vi "AlAs_GaAs_SL3.vi"(2 "Debug Mode":bool, 3 "Elapsed Time (s)":dbl, 4 "State":enum16{"Edit", "Start", "Run", "End", "Idle"}(ring), 5 "Argument List In":string[](array[string])) -> (0 "Status Out":string, 1 "Argument List Out":string[](array[string]))   [LabVIEW 2011]
doc: "This VI oscillates the flow of Gallium in a square wave according to the \"Period\" and \"Amplitude\" parameters. See the API Programming Guide for more details."
panel:
  out "tTot(s)":dbl
  in  "periods":dbl
  in  "tGa (s)":dbl
  in  "Ga flow (sccm)":dbl
  out "Timer":dbl
  out "Previous Time":dbl
  in  "tAl (s)":dbl
  in  "Al flow (sccm)":dbl
  in  "Cancel":bool
  in  "OK":bool
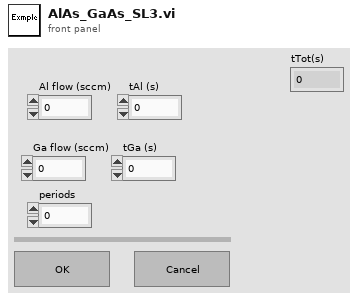
[diagram p1: front panel]
types:
  T1 = enum16{"Discrete", "Continuous", "Instantaneous"}
  T2 = enum32{"Invalid", "Default", "Floating", "Floating/Auto-Hide", "Modal"}
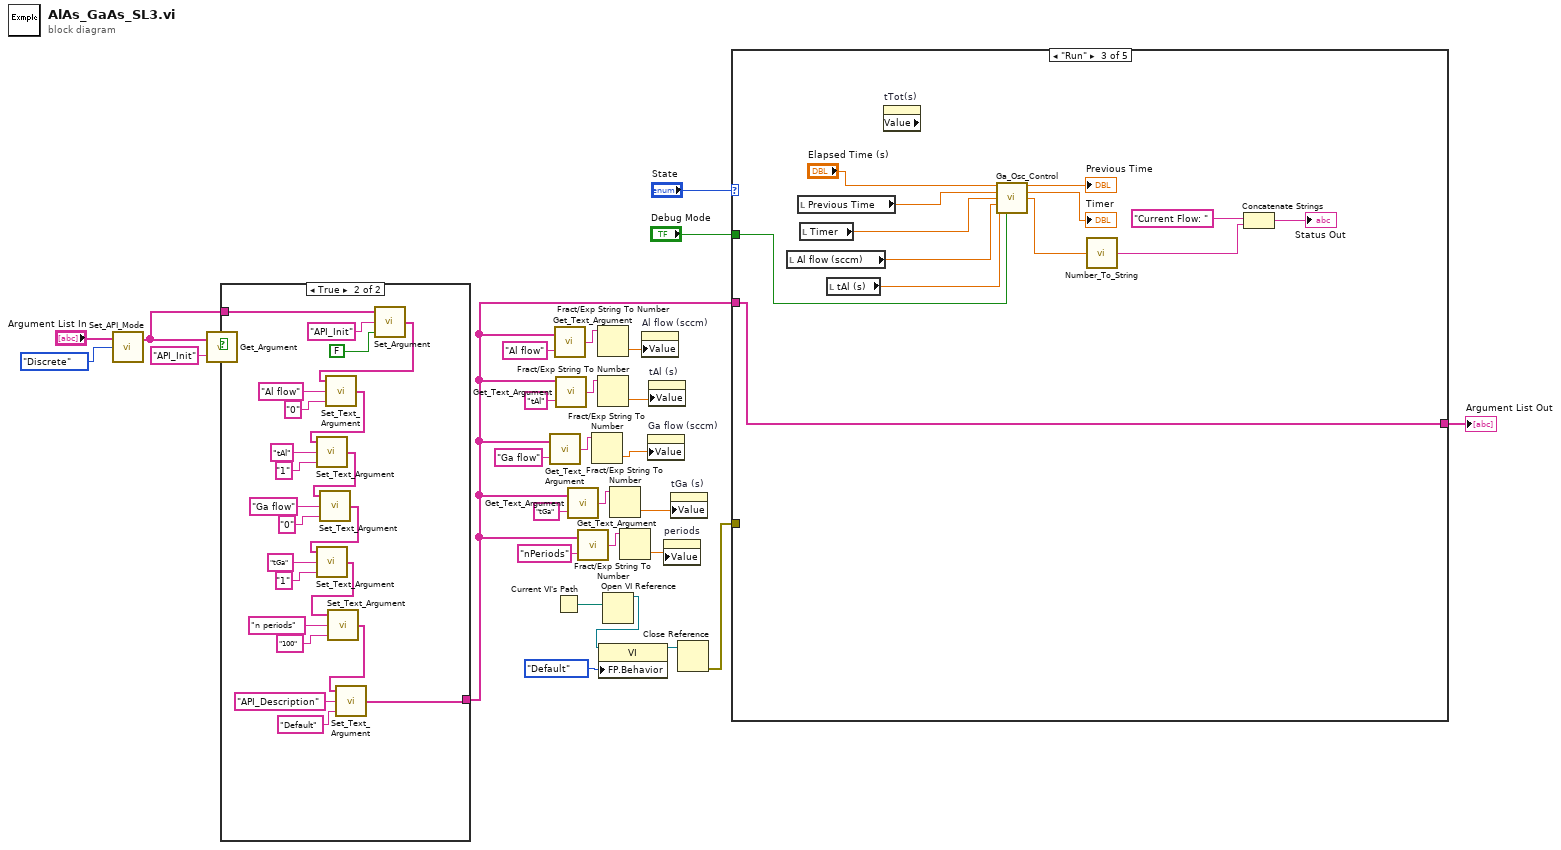
[diagram p0: block diagram]
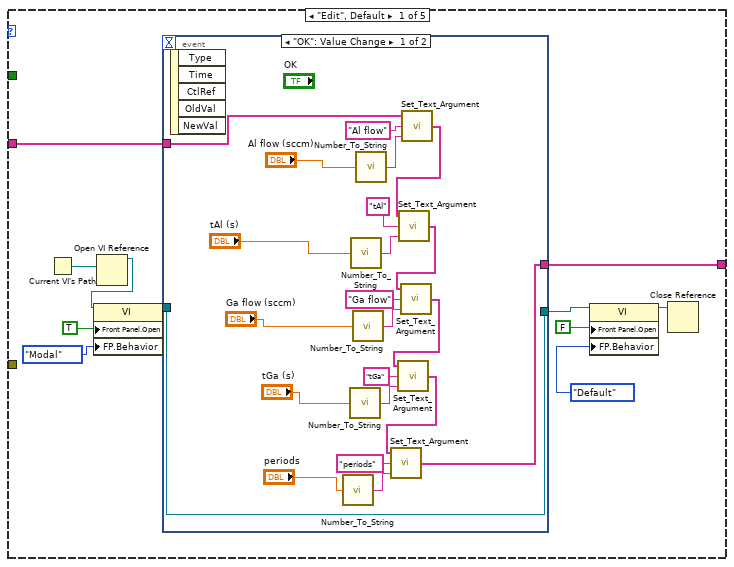
[diagram p3: hidden frame]
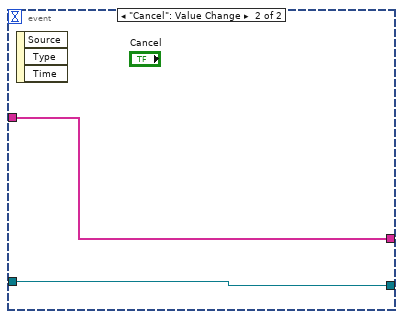
[diagram p4: hidden frame]
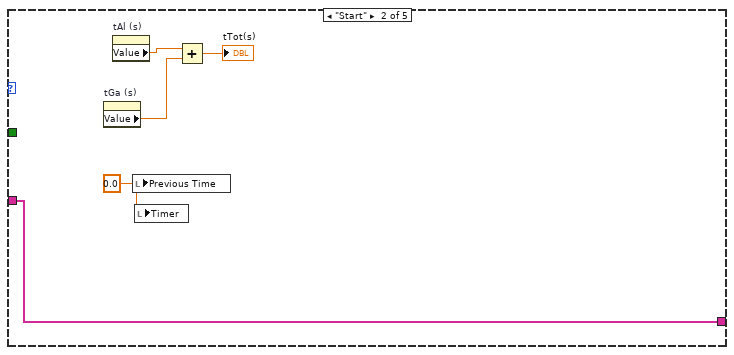
[diagram p5: hidden frame]
diagram:
  n1 = call "Set_API_Mode.vi"("API Mode"=T1."Discrete", "Argument List In"="Argument List In") -> ("Argument List Out"=w16:string[])  [unwired: 2 out]
  n2 = call "Get_Argument.vi"("Argument"="API_Init", "Argument List"=w16) -> ("Enabled"=w17:bool)
  n3 = case shown="True" w17 {
    tunnel: w16 -> [w30 w52]
    tunnel: [w30 w48] -> w6
    frame False {
    }
    frame True {
      n4 = call "Set_Argument.vi"("Enable"=FALSE, "Argument"="API_Init", "Argument List In"=w52) -> ("Argument List Out"=w31:string[])
      n5 = call "Set_Text_Argument.vi"("Text"="0", "Argument"="Al flow", "Argument List In"=w31) -> ("Argument List Out"=w32:string[])
      n6 = call "Set_Text_Argument.vi"("Text"="1", "Argument"="tAl", "Argument List In"=w32) -> ("Argument List Out"=w33:string[])
      n7 = call "Set_Text_Argument.vi"("Text"="0", "Argument"="Ga flow", "Argument List In"=w33) -> ("Argument List Out"=w34:string[])
      n8 = call "Set_Text_Argument.vi"("Text"="1", "Argument"="tGa", "Argument List In"=w34) -> ("Argument List Out"=w35:string[])
      n9 = call "Set_Text_Argument.vi"("Text"="100", "Argument"="n periods", "Argument List In"=w35) -> ("Argument List Out"=w36:string[])
      n10 = call "Set_Text_Argument.vi"("Text"="Default", "Argument"="API_Description", "Argument List In"=w36) -> ("Argument List Out"=w48:string[])
    }
  }
  n11 = call "Get_Text_Argument.vi"("Argument"="Ga flow", "Argument List"=w6) -> ("Text"=w11:string)
  n12 = Current VI's Path() -> (path=w25:path)
  n13 = call "Get_Text_Argument.vi"("Argument"="Al flow", "Argument List"=w6) -> ("Text"=w14:string)
  n14 = call "Get_Text_Argument.vi"("Argument"="tAl", "Argument List"=w6) -> ("Text"=w13:string)
  n15 = call "Get_Text_Argument.vi"("Argument"="tGa", "Argument List"=w6) -> ("Text"=w9:string)
  n16 = call "Get_Text_Argument.vi"("Argument"="nPeriods", "Argument List"=w6) -> ("Text"=w7:string)
  n17 = Fract/Exp String To Number(string=w11) -> (number=w3:dbl)  [unwired: 4 out]
  n18 = Fract/Exp String To Number(string=w14) -> (number=w5:dbl)  [unwired: 4 out]
  n19 = Fract/Exp String To Number(string=w13) -> (number=w4:dbl)  [unwired: 4 out]
  n20 = Open VI Reference(vi path=w25) -> (vi reference=w24:refnum<vi>)  [unwired: 1 in, 5 out]
  n21 = property class="VI"(reference=w24, "FP.Behavior"=T2."Default" ("Front Panel Window:Behavior")) -> (reference out=w22:refnum<vi>)  [unwired: 1 in, 1 out]
  n22 = Fract/Exp String To Number(string=w9) -> (number=w2:dbl)  [unwired: 4 out]
  n23 = Fract/Exp String To Number(string=w7) -> (number=w1:dbl)  [unwired: 4 out]
  n24 = property on="Al flow (sccm)" class="DigNum (strict)"("Value"=w5) -> ()  [unwired: 2 in, 2 out]
  n25 = property on="Ga flow (sccm)" class="DigNum (strict)"("Value"=w3) -> ()  [unwired: 2 in, 2 out]
  n26 = property on="tAl (s)" class="DigNum (strict)"("Value"=w4) -> ()  [unwired: 2 in, 2 out]
  n27 = property on="periods" class="DigNum (strict)"("Value"=w1) -> ()  [unwired: 2 in, 2 out]
  n28 = property on="tGa (s)" class="DigNum (strict)"("Value"=w2) -> ()  [unwired: 2 in, 2 out]
  n29 = Close Reference(reference=w22) -> (error out=w21:errorcluster)  [unwired: 1 in]
  n30 = case shown="\"Run\"" "State" {
    tunnel: [w63 w92 w103 w107 w108] -> w28
    tunnel: w6 -> [w62 w92 w103 w107 w108]
    tunnel: "Debug Mode" -> [_ _ w93 w106 _]
    tunnel: w21 -> [_ _ _ _ _]
    frame "Edit", Default {
      n31 = Current VI's Path() -> (path=w57:path)
      n32 = Open VI Reference(vi path=w57) -> (vi reference=w56:refnum<vi>)  [unwired: 1 in, 5 out]
      n33 = property class="VI"(reference=w56, "Front Panel.Open"=TRUE ("Front Panel Window:Open"), "FP.Behavior"=T2."Modal" ("Front Panel Window:Behavior")) -> (reference out=w60:refnum<vi>)  [unwired: 1 in, 1 out]
      n34 = event shown="[0] \"OK\": Value Change" {
        selector: _ -> [_ _]
        dyn-events: _ -> [_ _]
        timeout: _ -> [_ _]
        tunnel: w62 -> [w80 w86]
        tunnel: [w70 w86] -> w63
        tunnel: [w84 w87] -> w59
        tunnel: w60 -> [w84 w87]
        event "OK": Value Change {
          n35 = event-data() -> ()  [unwired: 6 out]
          n36 = call "Number_To_String.vi"("Number"="periods") -> ("String"=w72:string)
          n37 = call "Number_To_String.vi"("Number"="tGa (s)") -> ("String"=w74:string)
          n38 = call "Number_To_String.vi"("Number"="tAl (s)") -> ("String"=w81:string)
          n39 = call "Number_To_String.vi"("Number"="Ga flow (sccm)") -> ("String"=w76:string)
          n40 = call "Number_To_String.vi"("Number"="Al flow (sccm)") -> ("String"=w77:string)
          n41 = call "Set_Text_Argument.vi"("Text"=w77, "Argument"="Al flow" ("Text"), "Argument List In"=w80) -> ("Argument List Out"=w82:string[])
          n42 = call "Set_Text_Argument.vi"("Text"=w81, "Argument"="tAl", "Argument List In"=w82) -> ("Argument List Out"=w66:string[])
          n43 = call "Set_Text_Argument.vi"("Text"=w76, "Argument"="Ga flow", "Argument List In"=w66) -> ("Argument List Out"=w67:string[])
          n44 = call "Set_Text_Argument.vi"("Text"=w74, "Argument"="tGa", "Argument List In"=w67) -> ("Argument List Out"=w69:string[])
          n45 = call "Set_Text_Argument.vi"("Text"=w72, "Argument"="periods", "Argument List In"=w69) -> ("Argument List Out"=w70:string[])
        }
        event "Cancel": Value Change {
          n46 = event-data() -> ()  [unwired: 4 out]
        }
      }
      n47 = property class="VI"(reference=w59, "Front Panel.Open"=FALSE ("Front Panel Window:Open"), "FP.Behavior"=T2."Default" ("Front Panel Window:Behavior")) -> (reference out=w53:refnum<vi>)  [unwired: 1 in, 1 out]
      n48 = Close Reference(reference=w53) -> ()  [unwired: 1 in, 1 out]
    }
    frame "Start" {
      w91 = 0.0 ("Previous Time")
      n49 = property on="tGa (s)" class="DigNum (strict)"() -> ("Value"=w89:dbl)  [unwired: 2 in, 2 out]
      n50 = property on="tAl (s)" class="DigNum (strict)"() -> ("Value"=w90:dbl)  [unwired: 2 in, 2 out]
      n51 = local write "Previous Time"(w91) -> ()
      n52 = local write "Timer"(w91) -> ()
      n53 = Add(x=w90, y=w89) -> (x+y=→"tTot(s)":dbl)
    }
    frame "Run" {
      n54 = local read "Al flow (sccm)"() -> (w98:dbl)
      n55 = local read "Previous Time"() -> (w101:dbl)
      n56 = local read "Timer"() -> (w100:dbl)
      n57 = local read "tAl (s)"() -> (w97:dbl)
      n58 = property on="tTot(s)" class="DigNum (strict)" props=["Value"]() -> ()  [unwired: 2 in, 3 out]
      n59 = call "Ga_Osc_Control.vi"("Elapsed Time (s)"="Elapsed Time (s)", "Previous Time In"=w101, "Timer In"=w100, "Period"=w98, "Amplitude (sscm)"=w97, "Debug Mode"=w93) -> ("Previous Time Out"=→"Previous Time":dbl, "Timer Out"=→"Timer":dbl, "Flow"=w95:dbl)  [unwired: 7 out]
      n60 = call "Number_To_String.vi"("Number"=w95) -> ("String"=w94:string)
      n61 = Concatenate Strings("Current Flow: " ("string"), w94) -> (→"Status Out":string)
    }
    frame "End" {
      n62 = case shown="False" w106 {
        frame False {
        }
        frame True {
        }
      }
    }
    frame "Idle" {
    }
  }
  "Argument List Out" <- w28
